vi "GetAllDepsChain.vi"(7 "Skip Regenerate Linker Cache?":bool, 8 "error in (no error)":errorcluster, 10 "Library / Class Name":string, 11 "WorkSpace / Repo path":path) -> (0 "error out":errorcluster, 2 "All Dependency Chain":string, 3 "Dependency Chain []":string[](array[string]))   [LabVIEW 2019, in "Hawkeye.lvlib"]
uses:
  Hawkeye.lvlib
  <userlib>/_OpenG.lib/file/file.llb/File Exists - Scalar__ogtk.vi
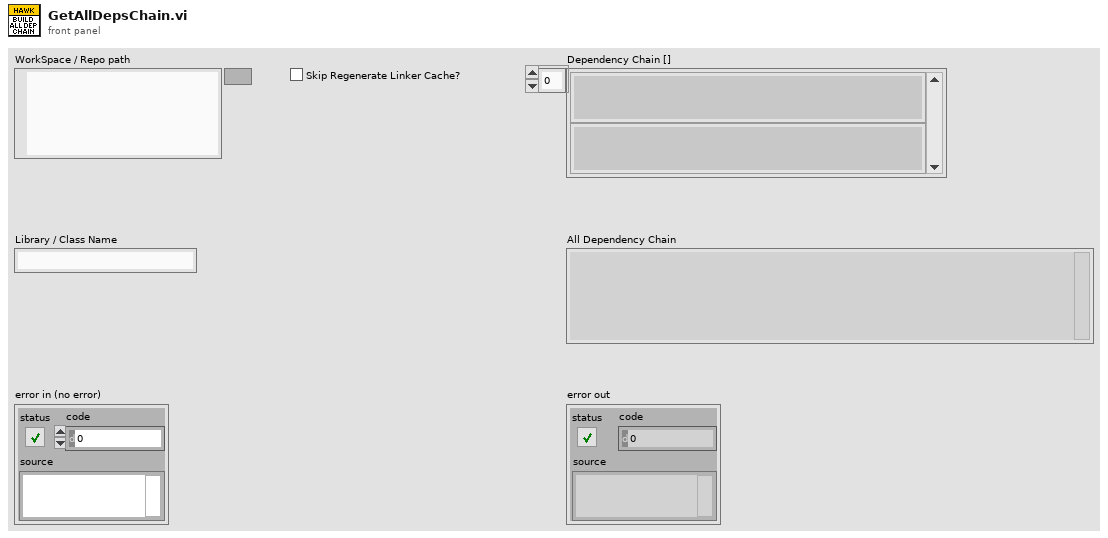
[diagram p1: front panel]
types:
  T1 = enum16{"open", "replace", "create", "open or create", "replace or create", "replace or create with confirmation"}
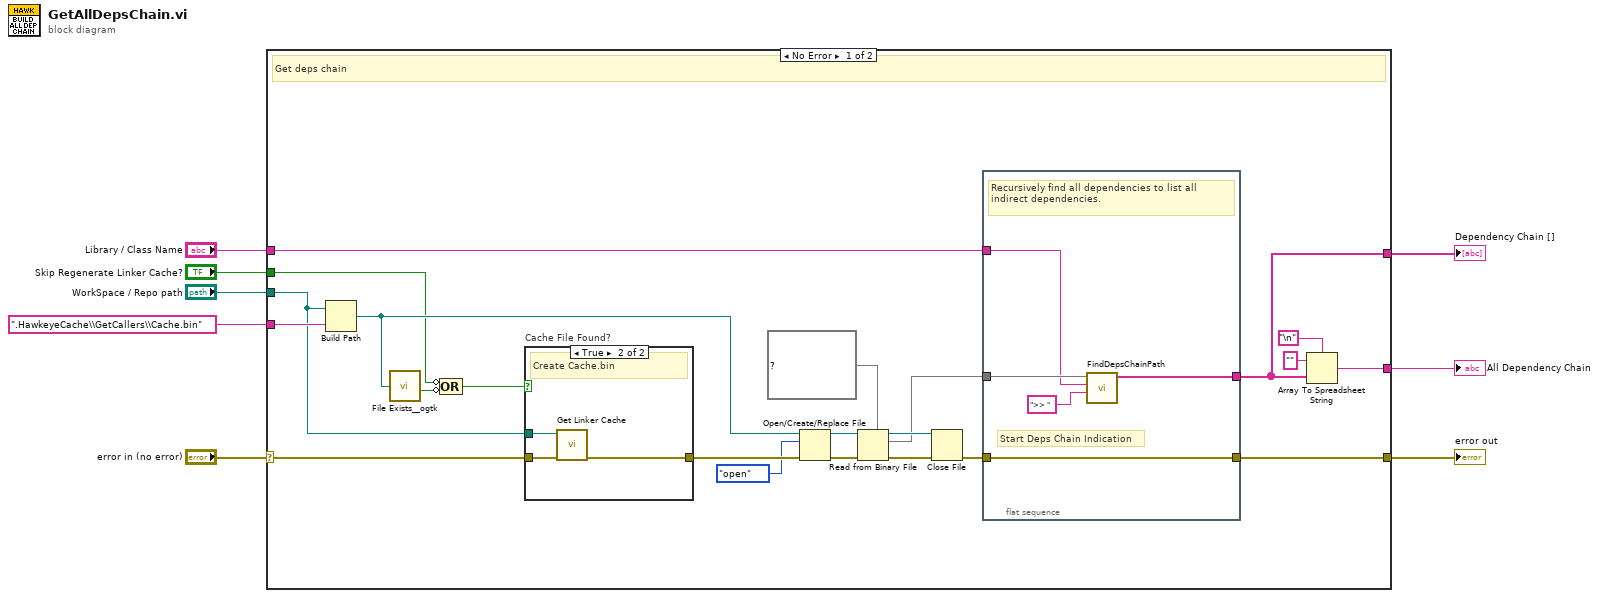
[diagram p0: block diagram]
diagram:
  n1 = case shown="No Error" "error in (no error)" {
    selector: "error in (no error)" -> [w17 w40]
    tunnel: [w28 _] -> w8
    tunnel: ".HawkeyeCache\\GetCallers\\Cache.bin" ("name or relative path") -> [w23 _]
    tunnel: [w21 w40] -> w6
    tunnel: "Library / Class Name" -> [w18 _]
    tunnel: "WorkSpace / Repo path" -> [w14 _]
    tunnel: [w12 _] -> w2
    tunnel: "Skip Regenerate Linker Cache?" -> [w9 _]
    frame No Error {
      # "Get deps chain"
      n2 = Build Path(base path=w14, name or relative path=w23) -> (appended path=w15:path)
      n3 = call-poly <userlib>:"File Exists__ogtk.vi"("file path"=w15) -> ("exists"=w11:bool)  [unwired: 6 in, 1 out]
      n4 = Compound Arithmetic op=OR(invert w9, invert w11) -> (w10:bool)
      n5 = case "Cache File Found?" shown="True" w10 {
        tunnel: w17 -> [w31 w34]
        tunnel: [w31 w33] -> w16
        tunnel: w14 -> [_ w32]
        frame False {
        }
        frame True {
          # "Create Cache.bin"
          n6 = call "Get Linker Cache.vi"("error in (no error)"=w34, "WorkSpace / Repo path"=w32) -> ("error out"=w33:errorcluster)  [unwired: 6 in, 3 out]
        }
      }
      n7 = Open/Create/Replace File(file path (use dialog)=w15, error in=w16, operation (0:open)=T1."open") -> (refnum out=w27:refnum<file>, error out=w24:errorcluster)  [unwired: 3 in, 1 out]
      n8 = Read from Binary File(5:map{string, string[]} {} ("Dependency Map"), 8:w24, 11:w27) -> (0:w25:errorcluster, 2:w19:map{string, string[]}, 3:w26:refnum<file>)  [unwired: 3 in, 1 out]
      n9 = Close File(refnum=w26, error in=w25) -> (error out=w20:errorcluster)  [unwired: 1 out]
      n10 = flat-sequence {
        tunnel: w18 -> [w37]
        tunnel: [w36] -> w12
        tunnel: w19 -> [w38]
        tunnel: [w39] -> w21
        tunnel: w20 -> [w39]
        frame #0 {
          # "Start Deps Chain Indication"
          # "Recursively find all dependencies to list all indirect dependencies."
          n11 = call "FindDepsChainPath.vi"("Dependency Path"=">> " ("Dependency"), "Current Dependency"=w37, "Dependency Map"=w38) -> ("Dependency Chain []"=w36:string[])  [unwired: 8 in]
        }
      }
      n12 = Array To Spreadsheet String(delimiter (Tab)="\n" ("Line Feed Constant"), array=w12, 3:"" ("format string")) -> (spreadsheet string=w28:string)
    }
    frame Error {
      # "error"
    }
  }
  "Dependency Chain []" <- w2
  "All Dependency Chain" <- w8
  "error out" <- w6
